vi "四旋翼姿态检测航行轨迹磁场校正上位机（加注释）.vi"() -> ()   [LabVIEW 2016]
uses:
  <vilib>/Utility/miscctls.llb/LVRGBAColorTypeDef.ctl
  <vilib>/Utility/miscctls.llb/LV3DPointTypeDef.ctl
  E:/LabVEIW/examples/Instrument IO/Serial/support/Serial - Settings.ctl
  E:/LabVEIW/examples/Instrument IO/Serial/support/Serial - XON-XOFF Characters.ctl
  E:/LabVEIW/examples/Instrument IO/Serial/support/Serial - ASCII Characters.ctl
  <vilib>/picture/3D Picture Control/Object/Create Object (name).vi
  <vilib>/picture/3D Picture Control/Object/Add Object (no reference).vi
  <vilib>/Instr/_visa.llb/VISA Configure Serial Port (Instr).vi
  <vilib>/picture/3D Picture Control/NI_3D Picture Control.lvlib
panel:
  in  "终止符":u8=10 format="%.0x"
  in  "终止符时结束写入？":bool=TRUE
  in  "VISA资源名称":refnum<visa-resource-name>="COM1"
  in  "XON/XOFF字符":T1={"XON"=enum."DC1", "XOFF"=enum."DC3"}
  in  "串口设置":T3={"波特率"=9600, "数据位"=8, "校验"=enum."None", "停止位"=10, "流控制"=0} {"流控制" items=["无"=0, "XON/XOFF"=1, "RTS/CTS"=2, "DTR/DSR"=4]; "停止位" items=["1.0"=10, "1.5"=15, "2.0"=20]; "数据位" min=5 max=8 step=1; "波特率" items=["75"=75, "110"=110, "134"=134, "150"=150, "300"=300, "600"=600, "1200"=1200, "1800"=1800, "2400"=2400, "4800"=4800, "7200"=7200, "9600"=9600, "14400"=14400, "19200"=19200, "28800"=28800, "38400"=38400, "56000"=56000, "57600"=57600, "115200"=115200, "128000"=128000, "230400"=230400]}
  in  "终止符时结束读取？":bool=TRUE
  out "响应":string
  out "θ":i32
  out "ψ":i32
  out "Φ":i32
  in  "字节总数":u32
  out "经度":i32
  out "纬度":i32
  out "磁场强度原始数据":i32
  in  "命令":string="*IDN?"
  in  "读取":bool
  in  "停止":bool
  in  "写入":bool
  in  "反光颜色":T4={"Red"=1.0, "Green"=1.0, "Blue"=1.0, "Alpha"=0.0} caption="场景光源反光颜色"
  in  "场景光源位置":T5
  in  "光源设置":u16(ring) items=["Inherit Value", "Off", "On"]
  out "四旋翼3D姿态模型":refnum<vi>(3d-picture)
  in  "自动投影模式":u16(ring) items=["None", "Perspective", "Orthographic"]
  in  "视角控制器:类型":u16(ring) items=["None", "Spherical", "Flying", "Oriented"]
  in  "背景色":T4 caption="三维图片背景色"
  in  "三维图片缩放":cluster{"X":sgl, "Y":sgl, "Z":sgl}
  out "连接的字符串":string
  in  "WebBrowser":refnum<k7>(container) caption="飞行轨迹"
  out "beforedata":dbl
  out "afterdata":dbl
  out "校正前磁场强度":dbl[](graph)
  out "校正后磁场强度":dbl[](graph)
  # "四旋翼姿态检测航行轨迹磁场矫正一体可视化化系统\n梁植源  孙一仆"
  # "串口配置"
  # "串口收发"
  # "数据处理"
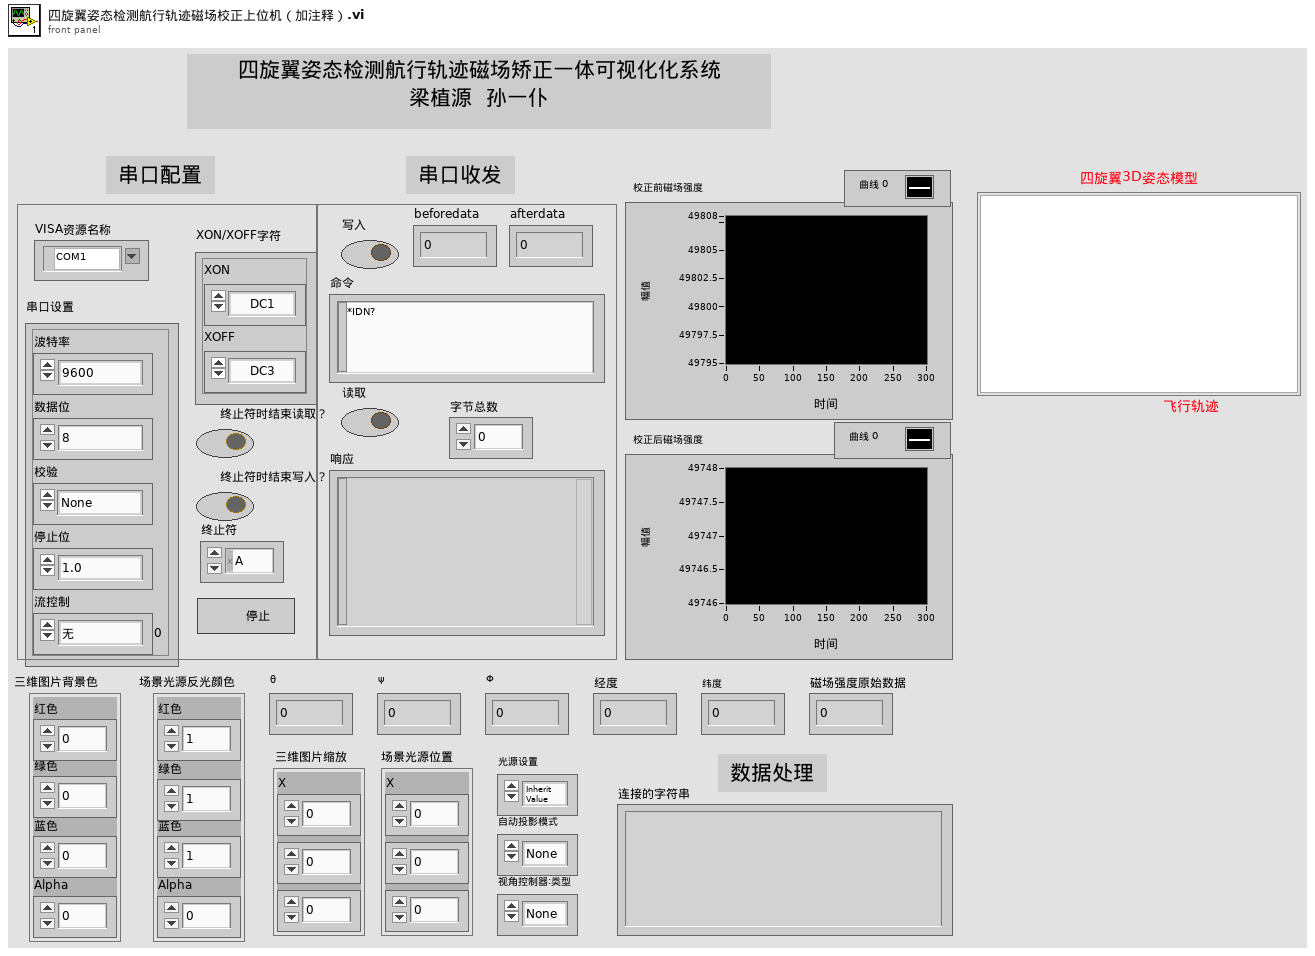
[diagram p1: front panel]
types:
  T1 = typedef "Serial - XON-XOFF Characters.ctl" = cluster{"XON":T2, "XOFF":T2}
  T2 = typedef "Serial - ASCII Characters.ctl" = enum16{"NUL", "SOH", "STX", "ETX", "EOT", "ENQ", "ACK", "BEL", "BS", "HT", "LF", "VT", "FF", "CR", "SO", "SI", "DLE", "DC1", "DC2", "DC3", "DC4", "NAK", "SYN", "ETB", "CAN", "EM", "SUB", "ESC", "FS", "GS", "RS", "US", "SP", "!", "\"", "#", "$", "%", "&", "'", "(", ")", "*", "+", ",", "- (-)", ".", "/", "0", "1", "2", "3", "4", "5", "6", "7", "8", "9", ":", ";", "<", "=", ">", "?", "@", "A", "B", "C", "D", "E", "F", "G", "H", "I", "J", "K", "L", "M", "N", "O", "P", "Q", "R", "S", "T", "U", "V", "W", "X", "Y", "Z", "[", "\\", "]", "^", "_", "`", "a", "b", "c", "d", "e", "f", "g", "h", "i", "j", "k", "l", "m", "n", "o", "p", "q", "r", "s", "t", "u", "v", "w", "x", "y", "z", "{", "|", "}", "~"}
  T3 = typedef "Serial - Settings.ctl" = cluster{"波特率":u32, "数据位":u16, "校验":enum16{"None", "Odd", "Even", "Mark", "Space"}, "停止位":u16, "流控制":u16}
  T4 = typedef "LVRGBAColorTypeDef.ctl" = cluster{"Red":sgl, "Green":sgl, "Blue":sgl, "Alpha":sgl}
  T5 = typedef "LV3DPointTypeDef.ctl" = cluster{"X":sgl, "Y":sgl, "Z":sgl}
  T6 = cluster{"Red":sgl, "Green":sgl, "Blue":sgl, "Alpha":sgl}
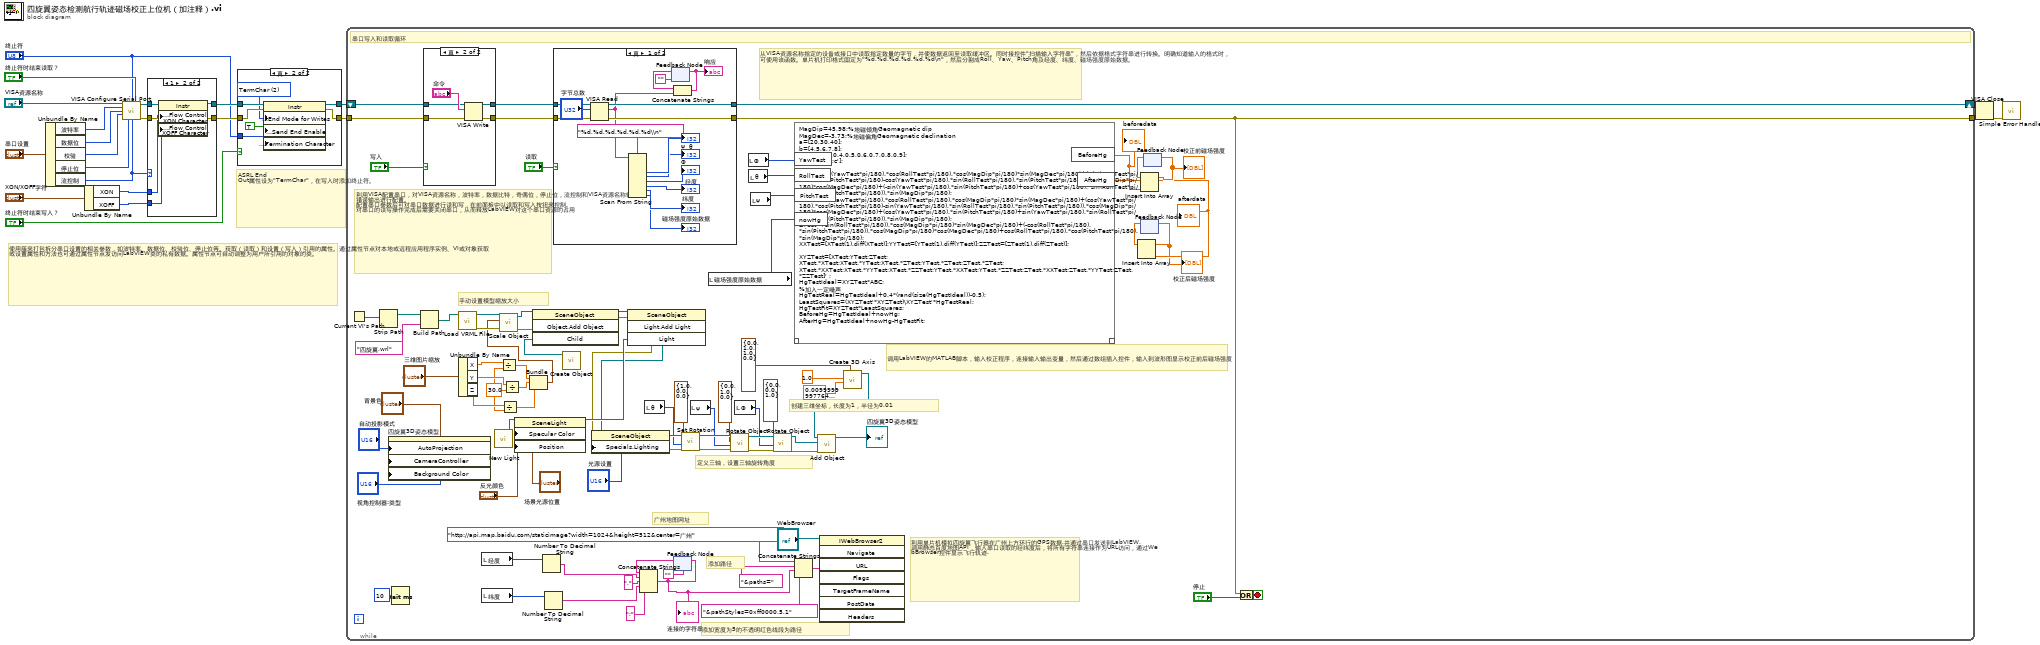
[diagram p0: block diagram]
diagram:
  # "使用簇来打包拆分串口设置的相关参数，如波特率、数据位、校验位、停止位等。获取（读取）和设置（写入）引用的属性。通过属性节点对本地或远程应用程序实例、VI或对象获取或设置属性和方法也可通过属性节点发访问LabVIEW类的私有数据。属性节点可自动调整为用户所引用的对象的类。"
  # "ASRL End Out属性设为\"TermChar\"，在写入时添加终止符。"
  n1 = Unbundle By Name("串口设置") -> ("波特率"=w5:u32, "数据位"=w4:u16, "校验"=w3:enum16{"None", "Odd", "Even", "Mark", "Space"}, "停止位"=w2:u16, "流控制"=w1:u16)
  n2 = Unbundle By Name("XON/XOFF字符") -> ("XON"=w14:T2, "XOFF"=w13:T2)
  n3 = call-poly "VISA Configure Serial Port"("VISA resource name"="VISA资源名称", "termination char\n(0xA = '\\n' = LF)"="终止符", "Enable Termination\nChar (T)"="终止符时结束读取？", "baud rate (9600)"=w5, "data bits (8)"=w4, "parity (0:none)"=w3, "stop bits (10: 1 bit)"=w2, "flow control (0:none)"=w1) -> ("VISA resource name out"=w19:refnum<visa-resource-name>, "error out"=w20:errorcluster)  [unwired: 2 in, 4 out]
  n4 = case shown="1" w1 {
    tunnel: [w23 w27] -> w12
    tunnel: [w24 w29] -> w10
    tunnel: w20 -> [w23 w28]
    tunnel: w19 -> [w24 w30]
    tunnel: w14 -> [_ w26]
    tunnel: w13 -> [_ w25]
    frame Default {
    }
    frame 1 {
      n5 = property class="Instr"(reference=w30, error in=w28, "Serial Settings:Flow Control XON Character"=w26, "Serial Settings:Flow Control XOFF Character"=w25) -> (reference out=w29:refnum<visa-resource-name>, error out=w27:errorcluster)
    }
  }
  n6 = case shown="真" "终止符时结束写入？" {
    tunnel: w10 -> [w31 w39]
    tunnel: w12 -> [w32 w38]
    tunnel: [w31 w37] -> w9
    tunnel: [w32 w36] -> w11
    tunnel: "终止符" -> [_ w34]
    frame False {
    }
    frame True {
      w35 = u16 2 items=["None", "LastBit", "TermChar", "Break"] ("Serial Settings:Serial End Mode for Writes")
      n7 = property class="Instr"(reference=w39, error in=w38, "Serial Settings:End Mode for Writes"=w35, "Message Based Settings:Send End Enable"=TRUE, "Message Based Settings:Termination Character"=w34) -> (reference out=w37:refnum<visa-resource-name>, error out=w36:errorcluster)
    }
  }
  n8 = while {
    shift-right: [w123] -> w15
    shift-left: w9 -> [w122]
    tunnel: w11 -> [w121]
    tunnel: [w115] -> w16
    stop <- w116 stop-if-true
    w68 = 30.0 ("y")
    # "广州地图网址"
    # "添加路径"
    # "添加宽度为5的不透明红色线段为路径"
    # "手动设置模型缩放大小"
    # "创建三维坐标，长度为1，半径为0.01"
    # "定义三轴，设置三轴旋转角度"
    # "利用单片机模拟四旋翼飞行器在广州上方环行的GPS数据,并通过串口发送到LabVIEW, 调用静态百度地图API，输入串口读取的经纬度后，将所有字符串连接作为URL访问，通过WebBrowser控件显示飞行轨迹."
    # "调用LabVIEW的MATLAB脚本，输入校正程序，连接输入输出变量，然后通过数组插入控件，输入到波形图显示校正前后磁场强度"
    # "从VISA资源名称指定的设备或接口中读取指定数量的字节，并使数据返回至读取缓冲区。同时接控件\"扫描输入字符串\"，然后依据格式字符串进行转换。明确知道输入的格式时，可使用该函数。单片机打印格式固定为\"%d,%d,%d,%d,%d,%d\\n\"，然后分割成Roll、Yaw、Pitch角及经度、纬度、磁场强度原始数据。"
    # "利用VISA配置串口，对VISA资源名称，波特率，数据比特，奇偶位，停止位，流控制和VISA资源名称输出和错误输出进行配置。\n配置串口参数后可对串口数据进行读和写，在前面板中以读取和写入按钮来控制。\n对串口的读写操作完成后需要关闭串口，从而释放LabVIEW对这个串口资源的占用"
    # "串口写入和读取循环"
    n9 = Current VI's Path() -> (path=w112:path)
    n10 = Strip Path(path=w112) -> (stripped path=w111:path)  [unwired: 1 out]
    n11 = property on="四旋翼3D姿态模型" class="SceneGraphDisp (严格)"("AutoProjection"="自动投影模式", "CameraController"="视角控制器:类型", "Background Color"="背景色") -> ()  [unwired: 2 in, 2 out]
    n12 = Wait (ms)(milliseconds to wait=u32 10) -> ()  [unwired: 1 out]
    n13 = Build Path(base path=w111, name or relative path="四旋翼.wrl" ("Name")) -> (appended path=w109:path)
    n14 = case shown="真" "写入" {
      tunnel: w122 -> [w125 w129]
      tunnel: w121 -> [w124 w128]
      tunnel: [w125 w127] -> w120
      tunnel: [w124 w126] -> w119
      frame False {
      }
      frame True {
        n15 = VISA Write(VISA resource name=w129, write buffer="命令", error in (no error)=w128) -> (VISA resource name out=w127:refnum<visa-resource-name>, error out=w126:errorcluster)  [unwired: 1 out]
      }
    }
    n16 = call <vilib>:"Load VRML File.vi"("Path"=w109) -> ("error out"=w75:errorcluster, "Scene:Read Scene File"=w76:refnum<vi>)  [unwired: 9 in]
    n17 = Unbundle By Name("三维图片缩放") -> ("X"=w71:sgl, "Y"=w70:sgl, "Z"=w69:sgl)
    n18 = local read "经度"() -> (w57:i32)
    n19 = local read "纬度"() -> (w56:i32)
    n20 = call <vilib>:"New Light.vi"() -> ("New Light Refnum"=w73:refnum<vi>)  [unwired: 10 in, 1 out]
    n21 = Divide(x=w71, y=w68) -> (x/y=w67:dbl)
    n22 = Divide(x=w69, y=w68) -> (x/y=w65:dbl)
    n23 = Divide(x=w70, y=w68) -> (x/y=w66:dbl)
    n24 = property class="SceneLight"(reference=w73, "Specular Color"="反光颜色", "Position"="场景光源位置") -> (reference out=w106:refnum<vi>)  [unwired: 1 in, 1 out]
    n25 = Bundle(w67, w66, w65) -> (w64:cluster{dbl, dbl, dbl})  [unwired: 1 in]
    n26 = call <vilib>:"Scale Object.vi"("error in (no error)"=w75, "Scale"=w64, "Scene.Object In"=w76) -> ("error out"=w77:errorcluster, "Scene.Object Out"=w78:refnum<vi>)  [unwired: 7 in]
    n27 = Number To Decimal String(number=w57) -> (decimal integer string=w55:string)  [unwired: 1 in]
    n28 = Number To Decimal String(number=w56) -> (decimal integer string=w54:string)  [unwired: 1 in]
    n29 = case shown="真" "读取" {
      tunnel: [w144 w148] -> w123
      tunnel: w120 -> [w146 w148]
      tunnel: [w143 w147] -> w115
      tunnel: w119 -> [w145 w147]
      frame True {
        n30 = VISA Read(VISA resource name=w146, byte count="字节总数", error in (no error)=w145) -> (VISA resource name out=w144:refnum<visa-resource-name>, read buffer=w137:string, error out=w143:errorcluster)  [unwired: 1 out]
        n31 = Scan From String(format string="%d,%d,%d,%d,%d,%d\\n" ("格式字符串"), input string=w137) -> (output 1=→"θ":i32, output 2=→"ψ":i32, output 3=→"Φ":i32, output 4=→"经度":i32, output 5=→"纬度":i32, output 6=→"磁场强度原始数据":i32)  [unwired: 8 in, 3 out]
        n32 = feedback #1("") -> (w142:string)
        n33 = Concatenate Strings(w142, w137) -> (w141:string)
        "响应" <- w141
        n34 = feedback-in #1(w141) -> ()
      }
      frame False {
      }
    }
    n35 = call-poly <vilib>:"Create Object.vi"() -> ("Scene:New Object"=w79:refnum<vi>)  [unwired: 10 in, 1 out]
    n36 = invoke class="SceneObject" method="Object.Add Object"(reference=w78, error in=w77, "Child"=w79) -> (reference out=w108:refnum<vi>, error out=w107:errorcluster)  [unwired: 1 in, 2 out]
    n37 = invoke class="SceneObject" method="Light.Add Light"(reference=w108, error in=w107, "Light"=w106) -> (reference out=w82:refnum<vi>, error out=w81:errorcluster)  [unwired: 1 in, 2 out]
    n38 = property on="属性节点" class="SceneObject"(reference=w82, error in=w81, "Specials.Lighting"="光源设置") -> (reference out=w104:refnum<vi>, error out=w103:errorcluster)
    n39 = local read "θ"() -> (w101:i32)
    n40 = feedback #2("") -> (w62:string)
    n41 = Concatenate Strings(w62, w55, "," ("字符串"), w54, ";" ("字符串")) -> (w50:string)
    "连接的字符串" <- w50
    n42 = feedback-in #2(w50) -> ()
    n43 = call <vilib>:"Set Rotation.vi"("error in (no error)"=w103, "Angle"=w101, "Axis"=cluster{"X":sgl, "Y":sgl, "Z":sgl} {"X"=1.0, "Y"=0.0, "Z"=0.0}, "Scene Object"=w104) -> ("error out"=w99:errorcluster, "Rotated Scene Object"=w100:refnum<vi>)  [unwired: 6 in]
    n44 = local read "ψ"() -> (w97:i32)
    n45 = local read "磁场强度原始数据"() -> (w46:i32)
    n46 = call <vilib>:"Rotate Object.vi"("error in (no error)"=w99, "Angle"=w97, "Axis"=cluster{"X":sgl, "Y":sgl, "Z":sgl} {"X"=0.0, "Y"=1.0, "Z"=0.0}, "Scene.Object In"=w100) -> ("error out"=w95:errorcluster, "Scene.Object Out"=w96:refnum<vi>)  [unwired: 6 in]
    n47 = local read "Φ"() -> (w93:i32)
    n48 = local read "Φ"() -> (w43:i32)
    n49 = local read "θ"() -> (w45:i32)
    n50 = local read "ψ"() -> (w44:i32)
    n51 = call <vilib>:"Rotate Object.vi"("error in (no error)"=w95, "Angle"=w93, "Axis"=cluster{"X":sgl, "Y":sgl, "Z":sgl} {"X"=0.0, "Y"=0.0, "Z"=1.0}, "Scene.Object In"=w96) -> ("error out"=w88:errorcluster, "Scene.Object Out"=w89:refnum<vi>)  [unwired: 6 in]
    n52 = script code="MagDip=45.98;%地磁倾角Geomagnetic dip\nMagDec=-3.73;%地磁偏角Geomagnetic declination\na=[20,30,40];\nb=[4,5,6,7,8];\nc=[0.2,0.3,0.4,0.5,0.6,0.7,0.8,0.9];\nABC=[a';b';c'];\n\nXTest=cos(YawTest*pi/180).*cos(RollTest*pi/180).*cos(MagDip*pi/180)*sin(MagDec*pi/180)+(-sin(YawTest*pi/180).*cos(PitchTest*pi/180)-cos(YawTest*pi/180).*sin(RollTest*pi/180).*sin(PitchTest*pi/180)).*cos(MagDip*pi/180)*cos(MagDec*pi/180)+(-sin(YawTest*pi/180).*sin(PitchTest*pi/180)+cos(YawTest*pi/180).*sin(RollTest*pi/180).*cos(PitchTest*pi/180)).*sin(MagDip*pi/180);\nYTest=sin(YawTest*pi/180).*cos(RollTest*pi/180).*cos(MagDip*pi/180)*sin(MagDec*pi/180)+(cos(YawTest*pi/180).*cos(PitchTest*pi/180)-sin(YawTest*pi/180).*sin(RollTest*pi/180).*sin(PitchTest*pi/180)).*cos(MagDip*pi/180)*cos(MagDec*pi/180)+(cos(YawTest*pi/180).*sin(PitchTest*pi/180)+sin(YawTest*pi/180).*sin(RollTest*pi/180).*cos(PitchTest*pi/180)).*sin(MagDip*pi/180);\nZTest=(-sin(RollTest*pi/180)).*cos(MagDip*pi/180)*sin(MagDec*pi/180)+(-cos(RollTest*pi/180).*sin(PitchTest*pi/180)).*cos(MagDip*pi/180)*cos(MagDec*pi/180)+cos(RollTest*pi/180).*cos(PitchTest*pi/180).*sin(MagDip*pi/180);\nXXTest=[XTest(1),diff(XTest)];YYTest=[YTest(1),diff(YTest)];ZZTest=[ZTest(1),diff(ZTest)];\n\nXYZTest=[XTest;YTest;ZTest;\nXTest.*XTest;XTest.*YTest;XTest.*ZTest;YTest.*ZTest;ZTest.*ZTest;\nXTest.*XXTest;XTest.*YYTest;XTest.*ZZTest;YTest.*XXTest;YTest.*ZZTest;ZTest.*XXTest;ZTest.*YYTest;ZTest.*ZZTest]' ;\nHgTestIdeal=XYZTest*ABC;\n%加入一定噪声\nHgTestReal=HgTestIdeal+0.4*(rand(size(HgTestIdeal))-0.5);\nLeastSquares=(XYZTest'*XYZTest)\\XYZTest'*HgTestReal;\nHgTestFit=XYZTest*LeastSquares;\nBeforeHg=HgTestIdeal+nowHg;\nAfterHg=HgTestIdeal+nowHg-HgTestFit;"("YawTest"=w43, "RollTest"=w45, "PitchTest"=w44, "nowHg"=w46) -> ("BeforeHg"=w48:dbl, "AfterHg"=w41:dbl)  [unwired: 1 in, 1 out]
    "beforedata" <- w48
    "afterdata" <- w41
    n53 = Concatenate Strings("http://api.map.baidu.com/staticimage?width=1024&height=512&center=广州" ("URL"), "&paths=" ("字符串"), w50, "&pathStyles=0xff0000,5,1" ("字符串")) -> (w59:string)
    n54 = invoke class="IWebBrowser2" method="Navigate"(reference="WebBrowser", "URL"=w59) -> ()  [unwired: 6 in, 8 out]
    n55 = call <vilib>:"Create 3D Axis.vi"("Color"=T6 {"Red"=0.0, "Green"=1.0, "Blue"=1.0, "Alpha"=0.0}, "Radius"=sgl 0.01, "Length"=sgl 1.0) -> ("New Object Refnum"=w83:refnum<vi>)  [unwired: 7 in, 1 out]
    n56 = call-poly <vilib>:"Add Object.vi"("error in (no error)"=w88, "New Object In"=w89, "Scene Object In"=w83) -> ("Scene Object Out"=→"四旋翼3D姿态模型":refnum<vi>)  [unwired: 7 in, 1 out]
    n57 = feedback #3() -> (w47:dbl[])  [unwired: 1 in]
    n58 = Insert Into Array(array=w47, new element=w41) -> (w40:dbl[])  [unwired: 1 in]
    "校正后磁场强度" <- w40
    n59 = feedback-in #3(w40) -> ()
    n60 = feedback #4() -> (w49:dbl[])  [unwired: 1 in]
    n61 = Insert Into Array(array=w49, new element=w48) -> (w42:dbl[])  [unwired: 1 in]
    "校正前磁场强度" <- w42
    n62 = feedback-in #4(w42) -> ()
    n63 = Or(x=w115, y="停止") -> (x .or. y?=w116:bool)
  }
  n64 = VISA Close(VISA resource name=w15, error in (no error)=w16) -> (error out=w17:errorcluster)
  n65 = call <vilib>:"Simple Error Handler.vi"("error in (no error)"=w17) -> ()  [unwired: 1 in, 8 out]
